vi "DSF.Engine.Transfer Group.Set Current Iteration.vi"(8 "error in (no error)":errorcluster, 10 "iteration":u64=1, 11 "Transfer Group in":refnum<class "DSF.Engine.Transfer Group.lvclass">) -> (0 "error out":errorcluster, 3 "Transfer Group out":refnum<class "DSF.Engine.Transfer Group.lvclass">)   [LabVIEW 2017, in "DSF.Engine.lvlib" / "DSF.Engine.Transfer Group.lvclass"]
uses:
  DSF.Engine.Transfer Group.lvclass
  DSF.Engine.Transfer Group.lvclass/DSF.Engine.Transfer Group.ctl
  Timing/DSF.Engine.Timing.lvclass
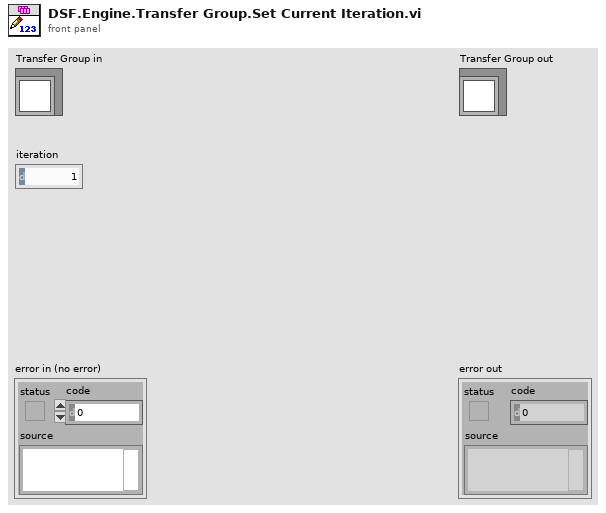
[diagram p1: front panel]
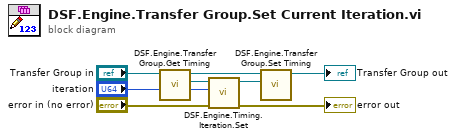
[diagram p0: block diagram]
diagram:
  n1 = call "DSF.Engine.Transfer Group.Get Timing.vi"("Transfer Group in"="Transfer Group in") -> ("Timing"=w7:refnum<class "DSF.Engine.Timing.lvclass">, "Transfer Group out"=w3:refnum<class "DSF.Engine.Transfer Group.lvclass">)  [unwired: 9 in]
  n2 = call "DSF.Engine.Timing.Iteration.Set.vi"("error in (no error)"="error in (no error)", "iteration"="iteration", "Timing in"=w7) -> ("error out"=→"error out":errorcluster, "Timing out"=w4:refnum<class "DSF.Engine.Timing.lvclass">)  [unwired: 7 in]
  n3 = call "DSF.Engine.Transfer Group.Set Timing.vi"("Timing"=w4, "Transfer Group in"=w3) -> ("Transfer Group out"=→"Transfer Group out":refnum<class "DSF.Engine.Transfer Group.lvclass">)  [unwired: 9 in]
